vi "Torque acquisition.vi"() -> ()   [LabVIEW 2018]
uses:
  <vilib>/Platform/TimedLoop/XDataNode/timing_clust.ctl
  <vilib>/Platform/TimedLoop/XDataNode/nitl_modes.ctl
  <vilib>/Platform/TimedLoop/XDataNode/wakeup.ctl
  <vilib>/rvi/Emulation/niFpgaGetClockAttributes.vi
  <vilib>/rvi/Emulation/niFpgaSctlEmulationGetInTimedLoop.vi
  <vilib>/rvi/Emulation/niFpgaEmulationReportErrorSimple.vi
  <vilib>/rvi/Emulation/niFpgaProcessEmulError.vi
  <vilib>/rvi/Emulation/niFpgaCriticalErrorInLSC.vi
  <vilib>/rvi/eio/common/nirviEmuTemplateMethod_errors.vi
  <vilib>/platform/TimedLoop/XDataNode/XDataNode.xnode
  <vilib>/eio/EIONode/EIONode.xnode
  <vilib>/Platform/TimedLoop/XDataNode/XDNodeRunTimeDep.lvlib
panel:
  in  "Stop calc":bool
  in  "STOP":bool
  out "Frequency (Hz)":u32
  out "pulses":u32
  in  "Teeth":u32=1
  in  "FPGA Clock":u32=40000000 format="%.0g"
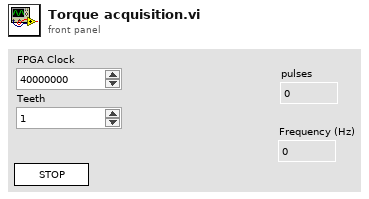
[diagram p1: front panel]
types:
  T1 = typedef "XDNodeRunTimeDep.lvlib/timing_clust.ctl" = cluster{"Expected End [f-1]":u64, "Actual End [f-1]":u64, "Finished Late? [f-1]":bool, "Expected End [i-1]":u64, "Actual End [i-1]":u64, "Finished Late? [i-1]":bool, "Expected Start [i]":u64, "Actual Start [i]":u64, "Expected Start [f]":u64, "Actual Start [f]":u64, "Source Name":string, "Structure Name":string, "Period":i64, "Deadline":i64, "Offset":i64, "Start":i64, "Priority":i32, "Timeout":i32, "Mode":T2, "Wakeup Reason":T3, "Error":errorcluster, "Source Type":string, "Secondary Source Type":string, "Global End Time":u64, "Global Start Time":u64, "Frame Duration":u64, "Iteration Duration":u64, "Assigned CPU":i32, "I/O Scan Engine Mode":u32}
  T2 = typedef "XDNodeRunTimeDep.lvlib/nitl_modes.ctl" = enum32{"No Change", "Process missed periods, maintain original phase", "Discard missed periods, maintain original phase", "Process missed periods, ignore original phase", "Discard missed periods, ignore original phase"}
  T3 = typedef "XDNodeRunTimeDep.lvlib/wakeup.ctl" = enum32{"Normal", "Aborted", "Asynchronous wakeup", "Timing source error", "Timed loop error", "Timeout"}
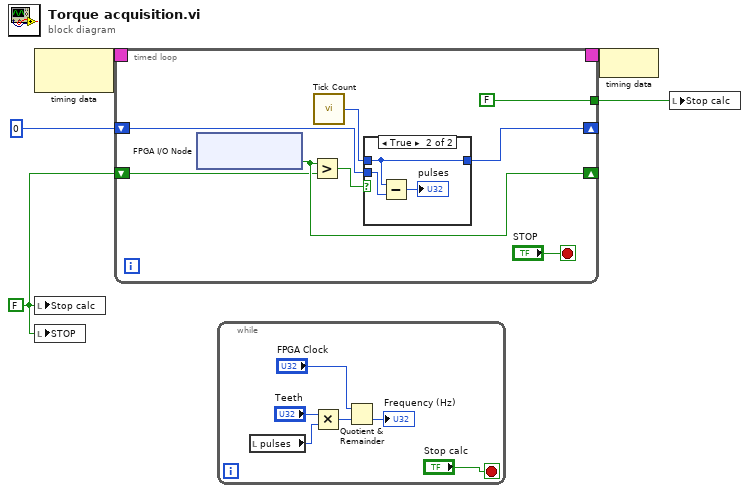
[diagram p0: block diagram]
diagram:
  w1 = FALSE
  n1 = node-c288() -> (w5:T1)  [unwired: 1 in]
  n2 = local write "Stop calc"(w1) -> ()
  n3 = local write "STOP"(w1) -> ()
  n4 = timed-loop {
    timing: w5 -> [_]
    timing-out: [_] -> w4
    shift-right: [w12] -> _
    shift-left: w1 -> [w6]
    shift-right: [w9] -> _
    shift-left: u32 0 ("Tick Count(Ticks)") -> [w11]
    tunnel: [FALSE ("Stop calc")] -> w2
    stop <- "STOP" stop-if-true
    n5 = xnode "FPGA I/O Node"() -> ("Mod8/DIO5"=w12:bool)  [unwired: 1 in, 1 out]
    n6 = Greater?(x=w12, y=w6) -> (0:w13:bool)
    n7 = call "Tick Count"() -> ("Tick Count(Ticks)"=w10:u32)
    n8 = case shown="True" w13 {
      tunnel: w11 -> [w14 w17]
      tunnel: w10 -> [_ w16]
      tunnel: [w14 w16] -> w9
      frame False {
      }
      frame True {
        n9 = Subtract(x=w16, y=w17) -> (x-y=→"pulses":u32)
      }
    }
  }
  n10 = while {
    stop <- "Stop calc" stop-if-true
    n11 = local read "pulses"() -> (w24:u32)
    n12 = Multiply(x="Teeth", y=w24) -> (x*y=w22:u32)
    n13 = Quotient & Remainder(x="FPGA Clock", y=w22) -> (floor(x/y)=→"Frequency (Hz)":u32)  [unwired: 1 out]
  }
  n14 = node-c288(w4) -> ()
  n15 = local write "Stop calc"(w2) -> ()
